vi "Parse DNS-SD Response.vi"(11 "response":T2 {"header"."response code" items=["NoError"=0, "FormErr"=1, "ServFail"=2, "NXDomain"=3, "NotImp"=4, "Refused"=5, "YXDomain"=6, "YXRRSet"=7, "NXRRSet"=8, "NotAuth"=9, "NotZone"=10, "DSOTYPENI"=11, "BADVERS/BADSIG"=16, "BADKEY"=17, "BADTIME"=18, "BADMODE"=19, "BADNAME"=20, "BADALG"=21, "BADTRUNC"=22, "BADCOOKIE"=23]; "header"."opcode" items=["Query"=0, "IQuery"=1, "Status"=2, "Notify"=4, "Update"=5, "DSO"=6]; "additional records"."class" items=["IN"=1, "CH"=3, "HS"=4]; "additional records"."type" items=["A"=1, "NS"=2, "MD"=3, "MF"=4, "CNAME"=5, "SOA"=6, "MB"=7, "MG"=8, "MR"=9, "NULL"=10, "WKS"=11, "PTR"=12, "HINFO"=13, "MINFO"=14, "MX"=15, "TXT"=16, "RP"=17, "AFSDB"=18, "X25"=19, "ISDN"=20, "RT"=21, "NSAP"=22, "NSAP-PTR"=23, "SIG"=24, "KEY"=25, "PX"=26, "GPOS"=27, "AAAA"=28, "LOC"=29, "NXT"=30, "EID"=31, "NIMLOC"=32, "SRV"=33, "ATMA"=34, "NAPTR"=35, "KX"=36, "CERT"=37, "A6"=38, "DNAME"=39, "SINK"=40, "OPT"=41, "APL"=42, "DS"=43, "SSHFP"=44, "IPSECKEY"=45, "RRSIG"=46, "NSEC"=47, "DNSKEY"=48, "DHCID"=49, "NSEC3"=50, "NSEC3PARAM"=51, "TLSA"=52, "SMIMEA"=53, "HIP"=55, "NINFO"=56, "RKEY"=57, "TALINK"=58, "CDS"=59, "CDNSKEY"=60, "OPENPGPKEY"=61, "CSYNC"=62, "ZONEMD"=63, "SVCB"=64, "HTTPS"=65, "SPF"=99, "UINFO"=100, "UID"=101, "GID"=102, "UNSPEC"=103, "NID"=104, "L32"=105, "L64"=106, "LP"=107, "EUI48"=108, "EUI64"=109, "URI"=256, "CAA"=257, "AVC"=258, "DOA"=259, "AMTRELAY"=260, "TA"=32768, "DLV"=32769]; "authority records"."class" items=["IN"=1, "CH"=3, "HS"=4]; "authority records"."type" items=["A"=1, "NS"=2, "MD"=3, "MF"=4, "CNAME"=5, "SOA"=6, "MB"=7, "MG"=8, "MR"=9, "NULL"=10, "WKS"=11, "PTR"=12, "HINFO"=13, "MINFO"=14, "MX"=15, "TXT"=16, "RP"=17, "AFSDB"=18, "X25"=19, "ISDN"=20, "RT"=21, "NSAP"=22, "NSAP-PTR"=23, "SIG"=24, "KEY"=25, "PX"=26, "GPOS"=27, "AAAA"=28, "LOC"=29, "NXT"=30, "EID"=31, "NIMLOC"=32, "SRV"=33, "ATMA"=34, "NAPTR"=35, "KX"=36, "CERT"=37, "A6"=38, "DNAME"=39, "SINK"=40, "OPT"=41, "APL"=42, "DS"=43, "SSHFP"=44, "IPSECKEY"=45, "RRSIG"=46, "NSEC"=47, "DNSKEY"=48, "DHCID"=49, "NSEC3"=50, "NSEC3PARAM"=51, "TLSA"=52, "SMIMEA"=53, "HIP"=55, "NINFO"=56, "RKEY"=57, "TALINK"=58, "CDS"=59, "CDNSKEY"=60, "OPENPGPKEY"=61, "CSYNC"=62, "ZONEMD"=63, "SVCB"=64, "HTTPS"=65, "SPF"=99, "UINFO"=100, "UID"=101, "GID"=102, "UNSPEC"=103, "NID"=104, "L32"=105, "L64"=106, "LP"=107, "EUI48"=108, "EUI64"=109, "URI"=256, "CAA"=257, "AVC"=258, "DOA"=259, "AMTRELAY"=260, "TA"=32768, "DLV"=32769]; "answers"."class" items=["IN"=1, "CH"=3, "HS"=4]; "answers"."type" items=["A"=1, "NS"=2, "MD"=3, "MF"=4, "CNAME"=5, "SOA"=6, "MB"=7, "MG"=8, "MR"=9, "NULL"=10, "WKS"=11, "PTR"=12, "HINFO"=13, "MINFO"=14, "MX"=15, "TXT"=16, "RP"=17, "AFSDB"=18, "X25"=19, "ISDN"=20, "RT"=21, "NSAP"=22, "NSAP-PTR"=23, "SIG"=24, "KEY"=25, "PX"=26, "GPOS"=27, "AAAA"=28, "LOC"=29, "NXT"=30, "EID"=31, "NIMLOC"=32, "SRV"=33, "ATMA"=34, "NAPTR"=35, "KX"=36, "CERT"=37, "A6"=38, "DNAME"=39, "SINK"=40, "OPT"=41, "APL"=42, "DS"=43, "SSHFP"=44, "IPSECKEY"=45, "RRSIG"=46, "NSEC"=47, "DNSKEY"=48, "DHCID"=49, "NSEC3"=50, "NSEC3PARAM"=51, "TLSA"=52, "SMIMEA"=53, "HIP"=55, "NINFO"=56, "RKEY"=57, "TALINK"=58, "CDS"=59, "CDNSKEY"=60, "OPENPGPKEY"=61, "CSYNC"=62, "ZONEMD"=63, "SVCB"=64, "HTTPS"=65, "SPF"=99, "UINFO"=100, "UID"=101, "GID"=102, "UNSPEC"=103, "NID"=104, "L32"=105, "L64"=106, "LP"=107, "EUI48"=108, "EUI64"=109, "URI"=256, "CAA"=257, "AVC"=258, "DOA"=259, "AMTRELAY"=260, "TA"=32768, "DLV"=32769]}) -> (3 "service instance":T1)   [LabVIEW 2015, in "PL DNS Client.lvlib"]
doc: "Parses DNS Service Discovery <b>response</b> and returns <b>service instance information</b>"
uses:
  PL DNS Client.lvlib
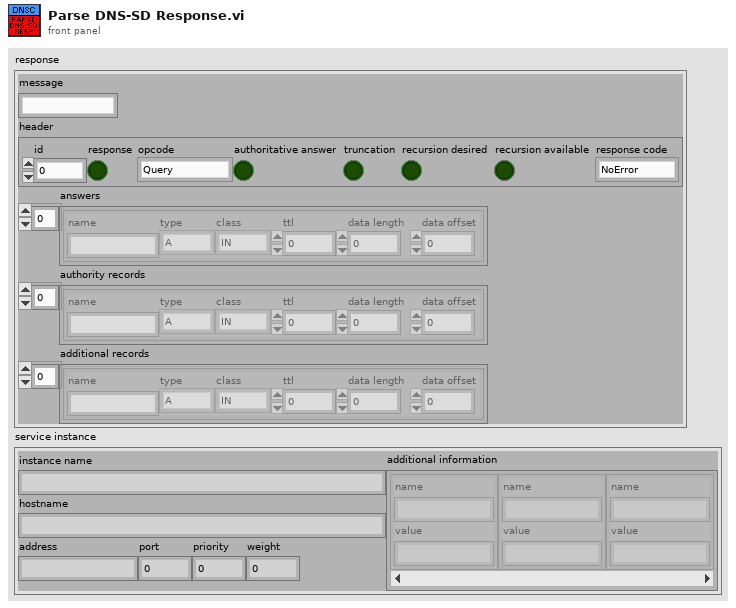
[diagram p1: front panel]
types:
  T1 = cluster{"instance name":string, "hostname":string, "address":string, "port":u16, "priority":u16, "weight":u16, "additional information":cluster{"name":string, "value":string}[]}
  T2 = cluster{"message":string, "header":cluster{"id":u16, "response":bool, "opcode":u8, "authoritative answer":bool, "truncation":bool, "recursion desired":bool, "recursion available":bool, "response code":u16}, "answers":cluster{"name":string, "type":u16, "class":u16, "ttl":u32, "data length":u16, "data offset":u16}[], "authority records":cluster{"name":string, "type":u16, "class":u16, "ttl":u32, "data length":u16, "data offset":u16}[], "additional records":cluster{"name":string, "type":u16, "class":u16, "ttl":u32, "data length":u16, "data offset":u16}[]}
  T3 = cluster{"name":string, "type":u16, "class":u16, "ttl":u32, "data length":u16, "data offset":u16}[]
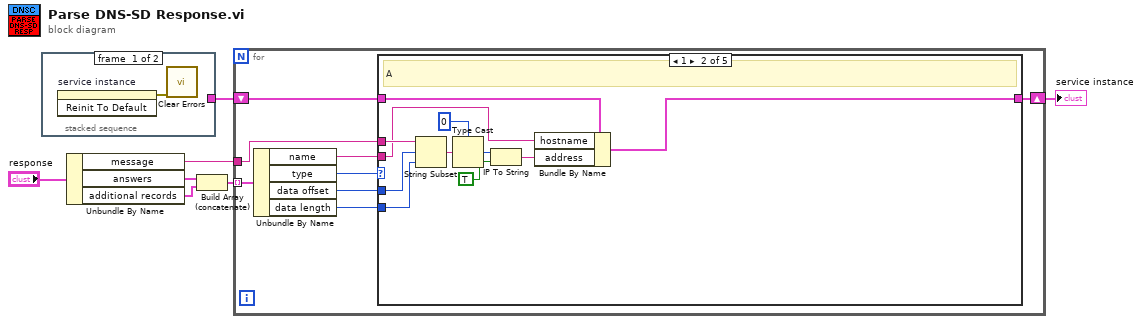
[diagram p0: block diagram]
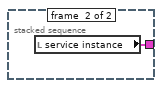
[diagram p2: hidden frame]
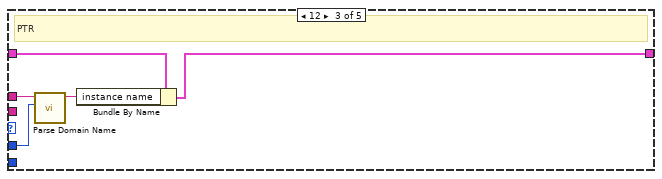
[diagram p4: hidden frame]
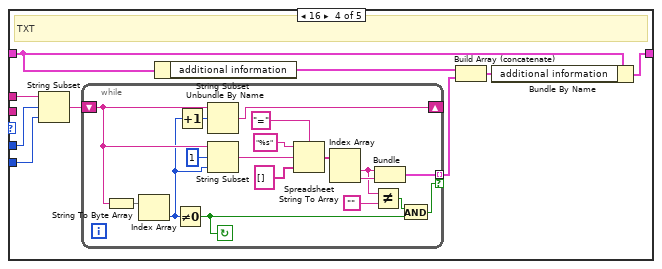
[diagram p5: hidden frame]
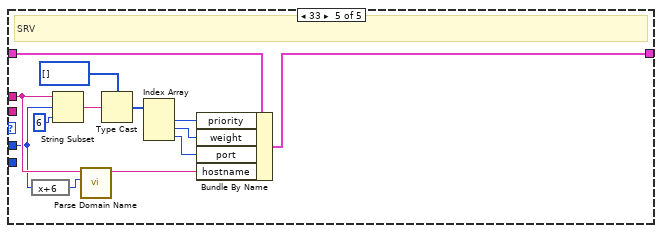
[diagram p6: hidden frame]
diagram:
  n1 = stacked-sequence {
    tunnel: [_ w9] -> w3
    frame #0 {
      n2 = invoke on="service instance" class="Clust (strict)" method="Reinit To Default"() -> (error out=w8:errorcluster)  [unwired: 3 in, 2 out]
      n3 = call <vilib>:"Clear Errors.vi"("error in (no error)"=w8) -> ()  [unwired: 5 in, 2 out]
    }
    frame #1 {
      n4 = local read "service instance"() -> (w9:T1)
    }
  }
  n5 = Unbundle By Name("response") -> ("message"=w6:string, "answers"=w7:T3, "additional records"=w4:T3)
  n6 = Build Array (concatenate)(w7, w4) -> (w5:T3)
  n7 = for {
    tunnel: w5 -> [w17] mode=indexing
    tunnel: w6 -> [w13]
    shift-right: [w12] -> w1
    shift-left: w3 -> [w16]
    n8 = Unbundle By Name(w17) -> ("name"=w14:string, "type"=w15:u16, "data offset"=w11:u16, "data length"=w10:u16)
    n9 = case shown="1" w15 {
      tunnel: w16 -> [w18 w25 w32 w39 w74]
      tunnel: w14 -> [_ w19 _ _ _]
      tunnel: w13 -> [_ w20 w34 w43 w65]
      tunnel: [w18 w23 w31 w35 w69] -> w12
      tunnel: w11 -> [_ w22 w33 w42 w64]
      tunnel: w10 -> [_ w21 _ w41 _]
      frame 0, Default {
      }
      frame 1 {
        # "A"
        n10 = String Subset(string=w20, offset (0)=w22, length (rest)=w21) -> (substring=w27:string)
        n11 = Type Cast(type=u32 0 ("net address"), x=w27) -> (*(type *) &x=w29:u32)
        n12 = IP To String(1:TRUE ("dot notation? (F)"), 2:w29) -> (0:w24:string)
        n13 = Bundle By Name(cluster=w25, "hostname"=w19, "address"=w24) -> (w23:T1)
      }
      frame 12 {
        # "PTR"
        n14 = call "Parse Domain Name.vi"("domain name offset"=w33, "message"=w34) -> ("domain name"=w30:string)  [unwired: 8 in, 1 out]
        n15 = Bundle By Name(cluster=w32, "instance name"=w30) -> (w31:T1)
      }
      frame 16 {
        # "TXT"
        n16 = String Subset(string=w43, offset (0)=w42, length (rest)=w41) -> (substring=w40:string)
        n17 = while {
          shift-right: [w59] -> _
          shift-left: w40 -> [w58]
          tunnel: [w49] -> w36 mode=indexing if=w45
          stop <- w48 continue-if-true
          n18 = String To Byte Array(string=w58) -> (unsigned byte array=w61:u8[])
          n19 = Index Array(array=w61) -> (element=w56:u8)  [unwired: 1 in]
          n20 = Not Equal To 0?(x=w56) -> (x != 0?=w48:bool)
          n21 = Increment(x=w56) -> (x+1=w60:u8)
          n22 = String Subset(string=w58, offset (0)=w60) -> (substring=w59:string)  [unwired: 1 in]
          n23 = String Subset(string=w58, offset (0)=1, length (rest)=w56) -> (substring=w55:string)
          n24 = Spreadsheet String To Array(delimiter (Tab)="=", format string="%s", spreadsheet string=w55, array type (2D Dbl)=string[] []) -> (array=w51:string[])
          n25 = Index Array(array=w51) -> (element #1=w47:string, element #2=w50:string)  [unwired: 2 in]
          n26 = Not Equal?(x=w47, y="") -> (x != y?=w44:bool)
          n27 = Bundle(w47, w50) -> (w49:cluster{string, string})  [unwired: 1 in]
          n28 = And(x=w44, y=w48) -> (x .and. y?=w45:bool)
        }
        n29 = Unbundle By Name(w39) -> ("additional information"=w38:cluster{"name":string, "value":string}[])
        n30 = Build Array (concatenate)(w38, w36) -> (w37:cluster{"name":string, "value":string}[])
        n31 = Bundle By Name(cluster=w39, "additional information"=w37) -> (w35:T1)
      }
      frame 33 {
        # "SRV"
        n32 = expression code="x+6"(w64) -> (w63:u16)
        n33 = String Subset(string=w65, offset (0)=w64, length (rest)=6 ("length (rest)")) -> (substring=w72:string)
        n34 = call "Parse Domain Name.vi"("domain name offset"=w63, "message"=w65) -> ("domain name"=w62:string)  [unwired: 8 in, 1 out]
        n35 = Type Cast(type=u16[] [], x=w72) -> (*(type *) &x=w70:u16[])
        n36 = Index Array(array=w70) -> (element #1=w68:u16, element #2=w67:u16, element #3=w66:u16)  [unwired: 3 in]
        n37 = Bundle By Name(cluster=w74, "priority"=w68, "weight"=w67, "port"=w66, "hostname"=w62) -> (w69:T1)
      }
    }
  }
  "service instance" <- w1
